vi "ProcessDataFlow.vi"(7 "Qbus in":refnum<class "Qbus.lvclass">, 8 "error in (no error)":errorcluster, 9 "DataGroups ChannelStatus":T1[](array[typedef]), 10 "Data":T7, 11 "config in":T3) -> (0 "error out":errorcluster, 3 "config out":T3)   [LabVIEW 2017, in "McsaTestPanel.lvlib"]
uses:
  <vilib>/addons/InsightCM/Devices/Shared/Mcsa/McsaTestPanel/McsaTestPanel.lvlib
  <vilib>/addons/InsightCM/Devices/Shared/Mcsa/McsaTestPanel/controls/Configuration.ctl
  <vilib>/addons/InsightCM/Devices/Shared/Common/TestPanel/controls/Configuration.ctl
  <vilib>/addons/InsightCM/Devices/Shared/Common/TestPanel/controls/State.ctl
  <vilib>/addons/InsightCM/MessageBus/Base/controls/IRoutingSource.ctl
  <vilib>/addons/InsightCM/Devices/Shared/Common/DataFlow/controls/Data.ctl
  <vilib>/addons/InsightCM/Utilities/DataAccessors/controls/wfmSGL_DVR.ctl
  <vilib>/addons/PointValueMap/controls/PointMap.ctl
  <vilib>/addons/InsightCM/Devices/Shared/Common/DataFlow/controls/Type.ctl
  <vilib>/addons/Qbus/Qbus.lvclass
  <vilib>/addons/InsightCM/Devices/Shared/Mcsa/McsaTestPanel/controls/ChannelStatus.ctl
  <vilib>/addons/InsightCM/MessageBus/Base/controls/KeyValuePair.ctl
  <vilib>/addons/InsightCM/MessageBus/MessageLibrary/Device/controls/DeviceTestPanelGetDataSetForChannelResponseBody.ctl
  <vilib>/addons/InsightCM/MessageBus/Base/controls/DataSetByteData.ctl
  <vilib>/addons/InsightCM/Devices/Shared/Common/TestPanel/TestPanel.lvlib
  <vilib>/addons/InsightCM/Devices/Shared/Common/ServerComm/ServerComm.lvlib
  <vilib>/addons/PointValueMap/PointValueMap.lvlib
  <vilib>/addons/InsightCM/Devices/Shared/Common/DataFlow/DataFlow.lvlib
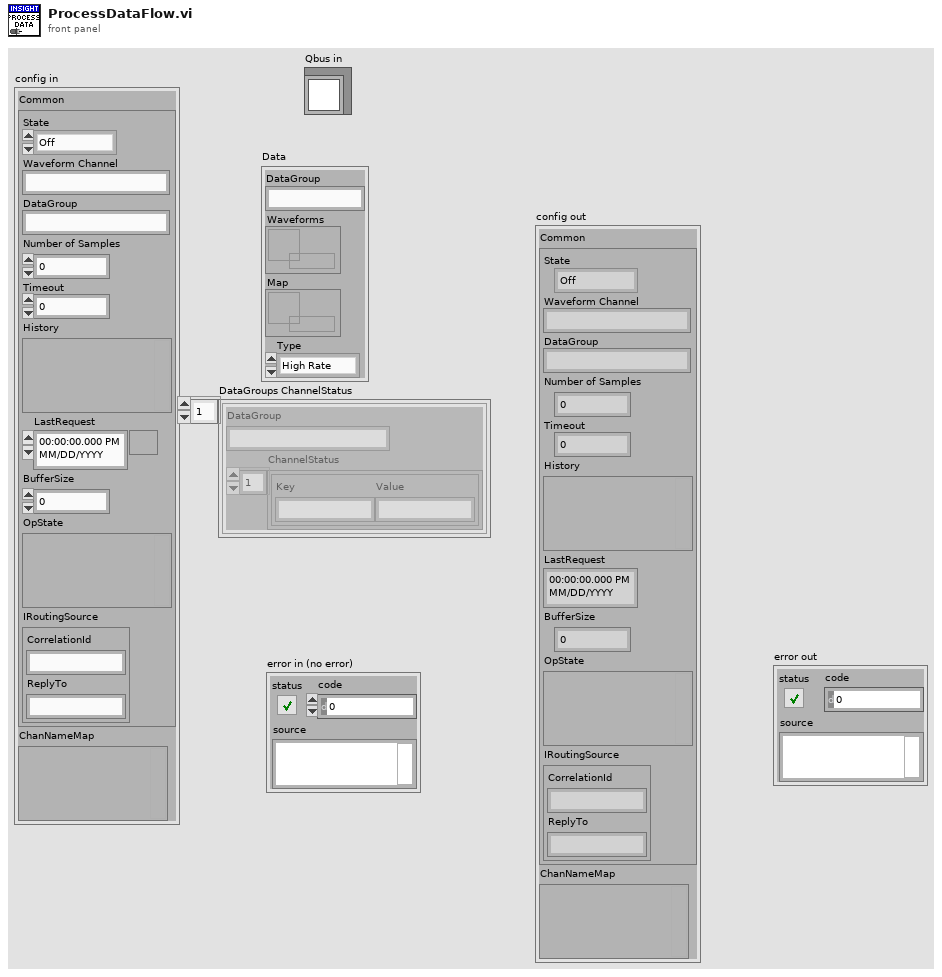
[diagram p1: front panel]
types:
  T1 = typedef "McsaTestPanel.lvlib/ChannelStatus.ctl" = cluster{"DataGroup":string, "ChannelStatus":T2[]}
  T2 = typedef "KeyValuePair.ctl" = cluster{"Key":string, "Value":string}
  T3 = typedef "McsaTestPanel.lvlib/Configuration.ctl" = cluster{"Common":T4, "ChanNameMap":variant}
  T4 = typedef "TestPanel.lvlib/Configuration.ctl" = cluster{"State":T5, "Waveform Channel":string, "DataGroup":string, "Number of Samples":i32, "Timeout":dbl, "History":variant, "LastRequest":timestamp, "BufferSize":i32, "OpState":variant, "IRoutingSource":T6}
  T5 = typedef "TestPanel.lvlib/State.ctl" = enum16{"Off", "On", "PendingValues", "PendingDataSet"}
  T6 = typedef "IRoutingSource.ctl" = cluster{"CorrelationId":string, "ReplyTo":string}
  T7 = typedef "DataFlow.lvlib/Data.ctl" = cluster{"DataGroup":string, "Waveforms":T8, "Map":T9, "Type":T10}
  T8 = typedef "wfmSGL_DVR.ctl" = refnum<data-value>
  T9 = typedef "PointValueMap.lvlib/PointMap.ctl" = refnum<data-value>
  T10 = typedef "DataFlow.lvlib/Type.ctl" = enum16{"High Rate", "Low Rate", "Burst Mode"}
  T11 = typedef "DeviceTestPanelGetDataSetForChannelResponseBody.ctl" = cluster{"DataSet":T12}
  T12 = typedef "DataSetByteData.ctl" = cluster{"Id":string, "DataEventId":string, "AssetNodeId":string, "Type":string, "T0":i64, "Props":T2[], "DataBase64":string}
  T13 = typedef "Message.ctl" = cluster{"Header":T14, "Body":u8[]}
  T14 = typedef "MessageHeader.ctl" = cluster{"MessageName":string, "Timestamp":i64, "CorrelationId":string, "ContentType":string, "RoutingKey":string, "Properties":T2[]}
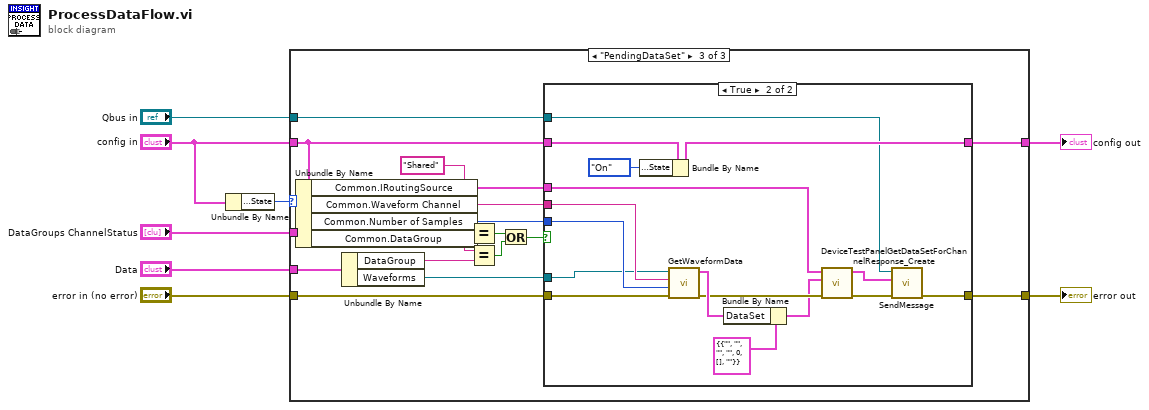
[diagram p0: block diagram]
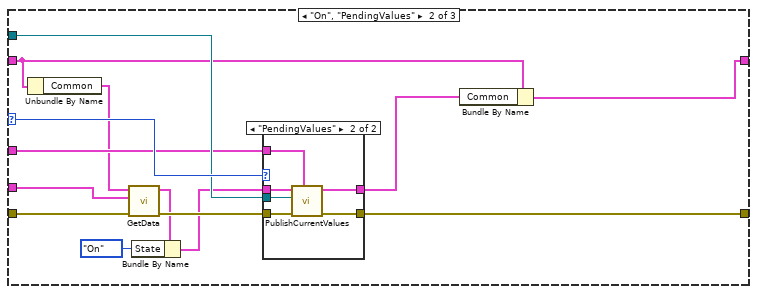
[diagram p3: hidden frame]
diagram:
  n1 = Unbundle By Name("config in") -> ("Common.State"=w8:T5)
  n2 = case shown="\"PendingDataSet\"" w8 {
    selector: w8 -> [_ w23 _]
    tunnel: "error in (no error)" -> [w10 w24 w48]
    tunnel: [w10 w22 w40] -> w3
    tunnel: "config in" -> [w9 w13 w43]
    tunnel: "Data" -> [_ w19 w45]
    tunnel: [w9 w11 w42] -> w4
    tunnel: "Qbus in" -> [_ w21 w41]
    tunnel: "DataGroups ChannelStatus" -> [_ w20 _]
    frame "Off" {
    }
    frame "On", "PendingValues" {
      n3 = Unbundle By Name(w13) -> ("Common"=w14:T4)
      n4 = call <vilib>:"GetData.vi"("error in (no error)"=w24, "Data"=w19, "config in"=w14) -> ("error out"=w18:errorcluster, "config out"=w16:T4)  [unwired: 7 in]
      n5 = Bundle By Name(cluster=w16, "State"=State."On") -> (w15:T4)
      n6 = case shown="\"PendingValues\"" w23 {
        tunnel: w15 -> [w25 w29]
        tunnel: w18 -> [w26 w32]
        tunnel: [w26 w31] -> w22
        tunnel: [w25 w30] -> w12
        tunnel: w21 -> [_ w28]
        tunnel: w20 -> [_ w27]
        frame Default {
        }
        frame "PendingValues" {
          n7 = call <vilib>:"PublishCurrentValues.vi"("DataGroups ChannelStatus"=w27, "error in (no error)"=w32, "Qbus in"=w28, "config in"=w29) -> ("error out"=w31:errorcluster, "config out"=w30:T4)  [unwired: 6 in]
        }
      }
      n8 = Bundle By Name(cluster=w13, "Common"=w12) -> (w11:T3)
    }
    frame "PendingDataSet" {
      n9 = Unbundle By Name(w43) -> ("Common.IRoutingSource"=w39:T6, "Common.Waveform Channel"=w47:string, "Common.Number of Samples"=w46:i32, "Common.DataGroup"=w37:string)
      n10 = Unbundle By Name(w45) -> ("DataGroup"=w38:string, "Waveforms"=w44:T8)
      n11 = Equal?(x="Shared", y=w37) -> (x = y?=w34:bool)
      n12 = Equal?(x=w37, y=w38) -> (x = y?=w35:bool)
      n13 = Or(x=w34, y=w35) -> (x .or. y?=w33:bool)
      n14 = case shown="True" w33 {
        tunnel: w48 -> [w50 w66]
        tunnel: w47 -> [_ w65]
        tunnel: w46 -> [_ w64]
        tunnel: w44 -> [_ w63]
        tunnel: w43 -> [w49 w62]
        tunnel: [w49 w60] -> w42
        tunnel: w41 -> [_ w56]
        tunnel: [w50 w57] -> w40
        tunnel: w39 -> [_ w52]
        frame False {
        }
        frame True {
          n15 = Bundle By Name(cluster=w62, "Common.State"=State."On" ("State")) -> (w60:T3)
          n16 = call <vilib>:"GetWaveformData.vi"("error in (no error)"=w66, "Number of Samples"=w64, "Current Channel"=w65, "Data Value Reference in"=w63) -> ("error out"=w55:errorcluster, "DataSet"=w59:T12)  [unwired: 6 in]
          n17 = Bundle By Name(cluster=T11 {"DataSet"={"Id"="", "DataEventId"="", "AssetNodeId"="", "Type"="", "T0"=0, "Props"=[], "DataBase64"=""}} ("DeviceTestPanelGetWaveformChannelResponse"), "DataSet"=w59) -> (w53:T11)
          n18 = call <vilib>:"DeviceTestPanelGetDataSetForChannelResponse_Create.vi"("error in (no error)"=w55, "DeviceTestPanelGetDataSetForChannelResponse"=w53, "IRoutingSource"=w52) -> ("error out"=w54:errorcluster, "Message"=w51:T13)  [unwired: 7 in]
          n19 = call <vilib>:"SendMessage.vi"("error in (no error)"=w54, "message"=w51, "Qbus in"=w56) -> ("error out"=w57:errorcluster)  [unwired: 7 in, 1 out]
        }
      }
    }
  }
  "error out" <- w3
  "config out" <- w4
